vi "Get PWM Channel Name.vi"(7 "PWM Channel Names":string[](array[string])=["A/PWM0", "A/PWM1", "A/PWM2", "B/PWM0", "B/PWM1", "B/PWM2", "C/PWM0", "C/PWM1"], 8 "Error In":errorcluster, 10 "PWM Channel Nums":u8[](array[numeric])) -> (0 "Error Out":errorcluster, 2 "PWM Channels":string[](array[string]))   [LabVIEW 2011, in "LMH-LINX.lvlib" / "myRIO.lvlib"]
doc: "Get PWM channel names (strings) from channel numbers."
uses:
  myRIO.lvlib
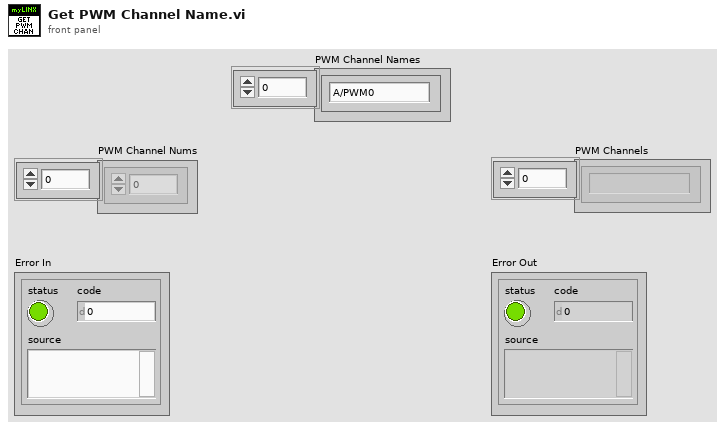
[diagram p1: front panel]
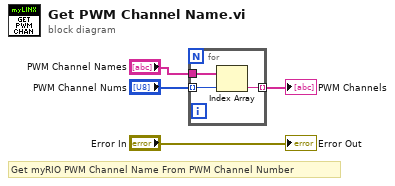
[diagram p0: block diagram]
diagram:
  # "Get myRIO PWM Channel Name From PWM Channel Number"
  n1 = for {
    tunnel: "PWM Channel Names" -> [w7]
    tunnel: "PWM Channel Nums" -> [w6] mode=indexing
    tunnel: [w5] -> w3 mode=indexing
    n2 = Index Array(array=w7, index=w6) -> (element=w5:string)
  }
  "PWM Channels" <- w3
  "Error Out" <- "Error In"
